vi "Get Digital Input.vi"(4 "error in (no error)":errorcluster, 6 "Axis In":i16, 7 "Controller Reference":refnum<k7>) -> (0 "error out":errorcluster, 1 "Boolean Input":bool, 2 "Axis Out":i16, 3 "Controller Reference out":refnum<k7>)   [LabVIEW 2015]
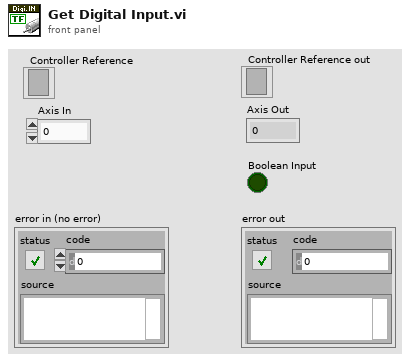
[diagram p1: front panel]
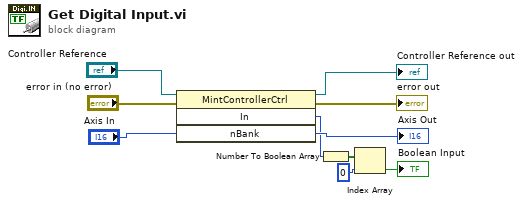
[diagram p0: block diagram]
diagram:
  n1 = invoke class="MintControllerCtrl" method="In"(reference="Controller Reference", error in="error in (no error)", "nBank"="Axis In") -> (reference out=→"Controller Reference out":refnum<k7>, error out=→"error out":errorcluster, "In"=w4:i32, "nBank"=→"Axis Out":i16)  [unwired: 1 in]
  n2 = Number To Boolean Array(number=w4) -> (Boolean array=w3:bool[])
  n3 = Index Array(array=w3, index=0) -> (element=→"Boolean Input":bool)
